vi "Run All Tests.vi"(7 "Open Caraya Results UI":bool, 8 "error in":errorcluster) -> (0 "error out":errorcluster)   [LabVIEW 2020]
uses:
  <vilib>/addons/_JKI Toolkits/Caraya/run-tests/Run Test (Scalar Path).vi
  <vilib>/addons/_JKI Toolkits/Caraya/Caraya.lvlib
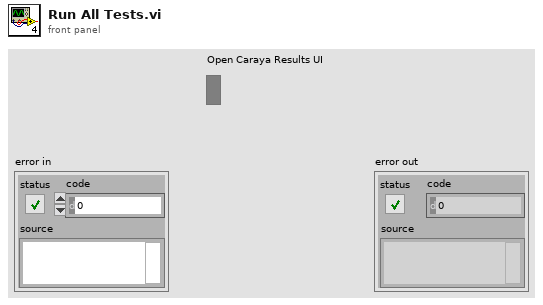
[diagram p1: front panel]
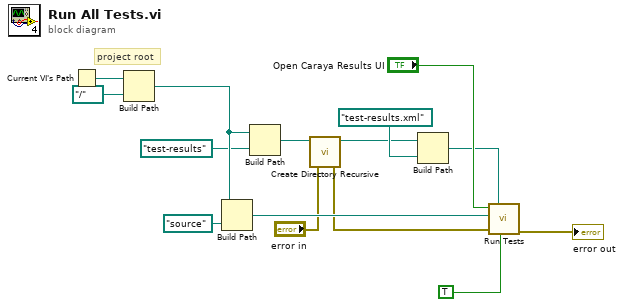
[diagram p0: block diagram]
diagram:
  # "project root"
  n1 = Current VI's Path() -> (path=w15:path)
  n2 = Build Path(base path=w15, name or relative path=path "../..") -> (appended path=w10:path)
  n3 = Build Path(base path=w10, name or relative path=path "source") -> (appended path=w11:path)
  n4 = Build Path(base path=w10, name or relative path=path "test-results") -> (appended path=w5:path)
  n5 = call <vilib>:"Create Directory Recursive.vi"("error in (no error)"="error in", "directory"=w5) -> ("error out"=w1:errorcluster, "directory copy"=w4:path)  [unwired: 3 in, 1 out]
  n6 = Build Path(base path=w4, name or relative path=path "test-results.xml") -> (appended path=w3:path)
  n7 = call-poly <vilib>:"Run Tests.vi"("Verbose"=TRUE, "Report Path"=w3, "error in"=w1, "Test Path"=w11, "Interactive (T)"="Open Caraya Results UI") -> ("error out"=→"error out":errorcluster)  [unwired: 5 in, 1 out]
